vi "Download Package List.vi"(8 "error in (no error)":errorcluster) -> (0 "error out":errorcluster, 3 "Packages":refnum<class "Package.lvclass">[](array[class]))   [LabVIEW 2017, in "GCentral API.lvlib"]
uses:
  GCentral API.lvlib
  Package/Package.lvclass
  Flatten To JSON Object/Flatten To JSON Object.lvclass
  C:/Users/de200256/Code/logmanoriginal/jsontext-object-serialization/vendor/drjdpowell-jsontext/LVClass Serializer/JSONtext LVClass Serializer.lvclass
  29494bb8-c315-48a3-8c75-717eca3f076a.vi
  <vilib>/JDP Science/JSONtext/JSON text to Variant.vi
  <vilib>/httpClient/LabVIEWHTTPClient.lvlib
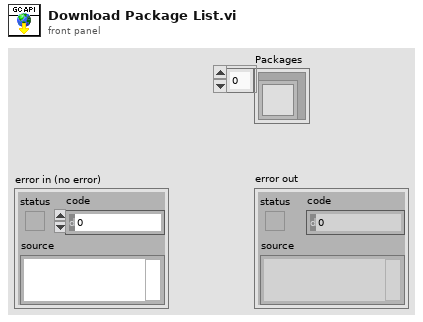
[diagram p1: front panel]
types:
  T1 = cluster{"packages":refnum<class "Package.lvclass">[]}
  T2 = typedef "LabVIEWHTTPClient.lvlib/ClientHandle.ctl" = refnum<k1>
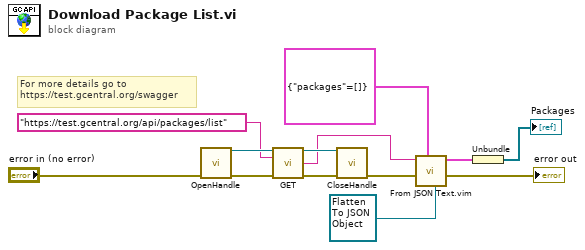
[diagram p0: block diagram]
diagram:
  # "For more details go to\nhttps://test.gcentral.org/swagger"
  n1 = call <vilib>:"OpenHandle.vi"("error in (no error)"="error in (no error)") -> ("client handle out"=w12:T2, "error out"=w13:errorcluster)  [unwired: 13 in]
  n2 = call <vilib>:"GET.vi"("client handle"=w12, "url"="https://test.gcentral.org/api/packages/list", "error in (no error)"=w13) -> ("client handle out"=w10:T2, "body"=w5:string, "error out"=w9:errorcluster)  [unwired: 9 in, 1 out]
  n3 = call <vilib>:"CloseHandle.vi"("client handle"=w10, "error in (no error)"=w9) -> ("error out"=w7:errorcluster)  [unwired: 13 in]
  n4 = call "From JSON Text.vim"("LVClass Serializer"=refnum<class "Flatten To JSON Object.lvclass"> refnum ("Flatten To JSON Object"), "Data Type and Default Value"=T1 {"packages"=[]}, "error in (no error)"=w7, "JSON"=w5) -> ("error out"=→"error out":errorcluster, "Data out"=w4:T1)  [unwired: 6 in]
  n5 = Unbundle(w4) -> ("packages"=→"Packages":refnum<class "Package.lvclass">[])
